vi "DataVIS_Preallocate 2D Intensity.vi"(8 "error in (no error)":errorcluster, 11 "dimension info":T2) -> (0 "error out":errorcluster, 3 "2D Intensity DVR":refnum<data-value>)   [LabVIEW 2016]
uses:
  <userlib>/LevyLab/Transport/SweepControl/Typedefs/Enum - Action.ctl
  <userlib>/LevyLab/Transport/SweepControl/SweepControl.lvclass
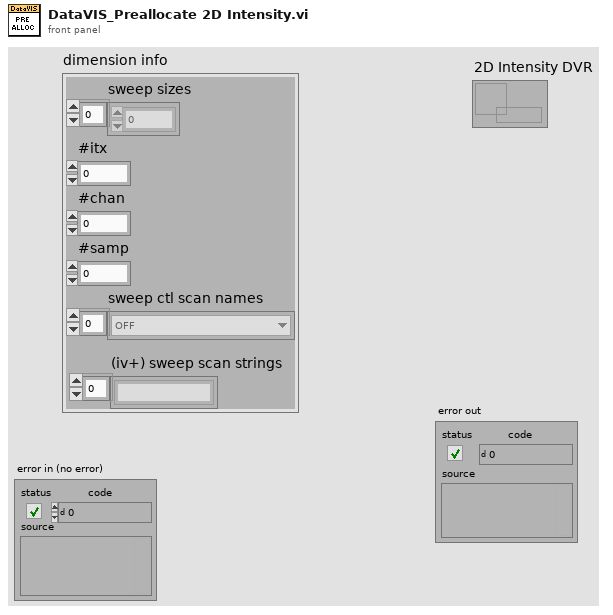
[diagram p1: front panel]
types:
  T1 = typedef "SweepControl.lvclass/Enum - Action.ctl" = enum16{"OFF", "DSA_Vamp", "DSA_freq", "DSA_Vsg1", "DSA_Vsg2", "DSA_Vsg3", "DAQ_Vbg", "B_Field", "Humidity", "Temp", "MW_freq1", "MW_freq2", "MW_amplitude1", "MW_amplitude2"}
  T2 = cluster{"sweep sizes":i32[], "#itx":i32, "#chan":i32, "#samp":i32, "sweep ctl scan names":T1[], "(iv+) sweep scan strings":string[]}
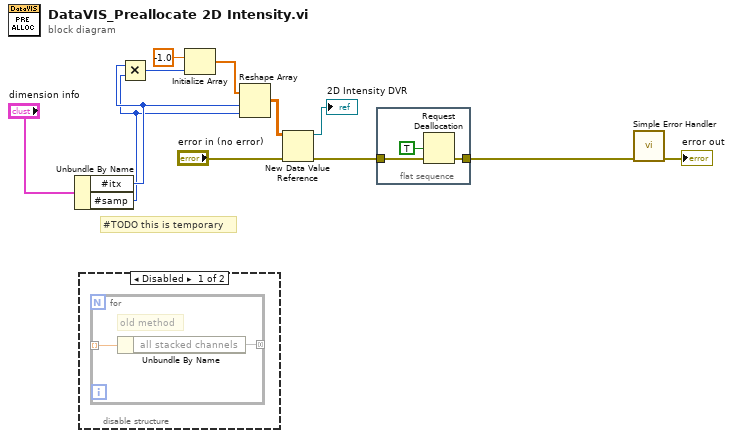
[diagram p0: block diagram]
diagram:
  # "#TODO this is temporary"
  n1 = Unbundle By Name("dimension info") -> ("#itx"=w3:i32, "#samp"=w2:i32)
  n2 = disable-structure shown="Disabled" {
    frame Disabled {
      n3 = for {
        tunnel: _ -> [w14] mode=indexing
        tunnel: [w13] -> _ mode=concatenating
        # "old method"
        n4 = Unbundle By Name(w14) -> ("all stacked channels"=w13)
      }
    }
    frame Enabled {
    }
  }
  n5 = Multiply(x=w3, y=w2) -> (x*y=w9:i32)
  n6 = Initialize Array(-1.0, w9) -> (w8:dbl[])
  n7 = Reshape Array(w8, w3, w2) -> (w7:dbl[][])
  n8 = New Data Value Reference(data value=w7, error in="error in (no error)") -> (data value reference=→"2D Intensity DVR":refnum<data-value>, error out=w5:errorcluster)
  n9 = flat-sequence {
    tunnel: w5 -> [w16]
    tunnel: [w16] -> w4
    frame #0 {
      n10 = Request Deallocation(TRUE ("flag")) -> ()
    }
  }
  n11 = call <vilib>:"Simple Error Handler.vi"("error in (no error)"=w4) -> ("error out"=→"error out":errorcluster)  [unwired: 4 in, 4 out]
